vi "test A_Set Hard Reset Status.vi"(11 "Test Case In":refnum<class "Test PCANBasic.lvclass">) -> (0 "error out":errorcluster, 3 "Test Case Out":refnum<class "Test PCANBasic.lvclass">)   [LabVIEW 2020, in "Test PCANBasic.lvclass"]
uses:
  Test PCANBasic.lvclass
  source/PCANBasic.lvlib
  Global PCAN Channel.vi
  Global PCAN Baudrate.vi
  <vilib>/Astemes/LUnit/Test Case.lvclass
  source/Set Hard Reset Status.vi
panel:
  # "Execute this first so that previois heavy bus errors are deleted"
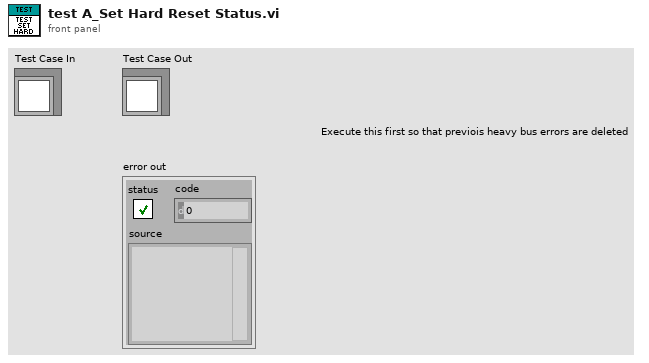
[diagram p1: front panel]
types:
  T1 = typedef "PCANBasic.lvlib/TPCANHandle.ctl" = u16
  T2 = typedef "PCANBasic.lvlib/PCAN Baud.ctl" = u16
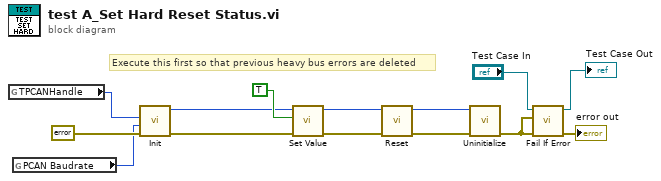
[diagram p0: block diagram]
diagram:
  # "Execute this first so that previous heavy bus errors are deleted"
  n1 = global read "Global PCAN Channel.vi" "TPCANHandle"() -> (w7:T1)
  n2 = global read "Global PCAN Baudrate.vi" "PCAN Baudrate"() -> (w5:T2)
  n3 = call "Init.vi"("error in"=errorcluster {"status"=FALSE, "code"=0, "source"=""}, "Baudrate"=w5, "Channel"=w7) -> ("error out"=w8:errorcluster, "TPCANHandle out"=w6:T1)  [unwired: 6 in, 1 out]
  n4 = call-poly "Set Value.vi"("error in"=w8, "Enable"=TRUE, "TPCANHandle in"=w6) -> ("error out"=w9:errorcluster, "TPCANHandle out"=w3:T1)  [unwired: 6 in, 1 out]
  n5 = call "Reset.vi"("error in"=w9, "TPCANHandle in"=w3) -> ("error out"=w4:errorcluster, "TPCANHandle out"=w2:T1)  [unwired: 7 in, 1 out]
  n6 = call "Uninitialize.vi"("error in"=w4, "TPCANHandle in"=w2) -> ("error out"=w1:errorcluster)  [unwired: 8 in, 1 out]
  n7 = call <vilib>:"Fail If Error.vi"("error in (no error)"=w1, "Assert error"=w1, "LUnit Test Case In"="Test Case In") -> ("error out"=→"error out":errorcluster, "LUnit Test Case Out"=→"Test Case Out":refnum<class "Test PCANBasic.lvclass">)  [unwired: 7 in]
